vi "Cycle RGB Colors.vi"(3 "Magnitude":dbl, 4 "Cycle Speed":i32=5, 5 "Iteration":i32, 6 "Cycle Colors?":bool) -> (0 "Blue Value":u8, 1 "Green Value":u8, 2 "Red Value":u8)   [LabVIEW 2011, in "LabVIEW Interface for Arduino.lvlib"]
doc: "Cycles through RGB colors and outputs the appropriate Red Green and Blue values scaled by the specified Magnitude."
uses:
  LabVIEW Interface for Arduino.lvlib
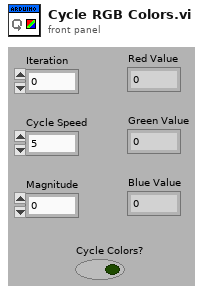
[diagram p1: front panel]
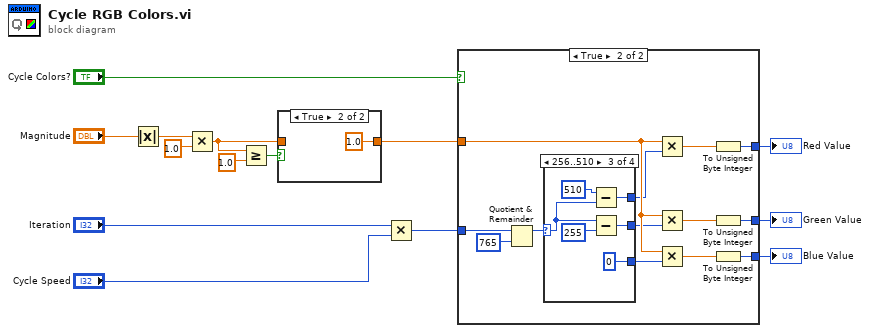
[diagram p0: block diagram]
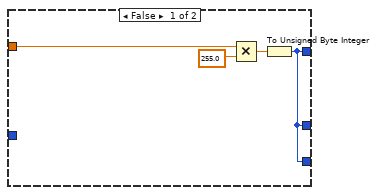
[diagram p2: hidden frame]
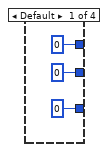
[diagram p3: hidden frame]
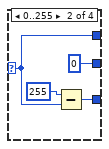
[diagram p4: hidden frame]
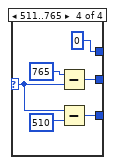
[diagram p5: hidden frame]
diagram:
  n1 = Absolute Value(x="Magnitude") -> (abs(x)=w1:dbl)
  n2 = Multiply(x=w1, y=1.0) -> (x*y=w5:dbl)
  n3 = Greater Or Equal?(x=w5, y=1.0) -> (x >= y?=w4:bool)
  n4 = case shown="True" w4 {
    tunnel: w5 -> [w15 _]
    tunnel: [w15 1.0 ("y")] -> w7
    frame False {
    }
    frame True {
    }
  }
  n5 = Multiply(x="Iteration", y="Cycle Speed") -> (x*y=w13:i32)
  n6 = case shown="True" "Cycle Colors?" {
    tunnel: w13 -> [_ w31]
    tunnel: w7 -> [w18 w30]
    tunnel: [w20 w23] -> w10
    tunnel: [w20 w22] -> w8
    tunnel: [w20 w21] -> w9
    frame False {
      n7 = Multiply(x=w18, y=255.0) -> (x*y=w17:dbl)
      n8 = To Unsigned Byte Integer(number=w17) -> (unsigned 8bit integer=w20:u8)
    }
    frame True {
      n9 = Quotient & Remainder(x=w31, y=765) -> (x-y*floor(x/y)=w33:i32)  [unwired: 1 out]
      n10 = case shown="256..510" w33 {
        selector: w33 -> [_ w40 w41 w48]
        tunnel: [0 ("y") w40 w44 0 ("y")] -> w29
        tunnel: [0 0 w45 w49] -> w28
        tunnel: [0 ("y") w38 u8 0 ("y") w50] -> w27
        frame Default {
        }
        frame 0..255 {
          n11 = Subtract(x=255, y=w40) -> (x-y=w38:i32)
        }
        frame 256..510 {
          n12 = Subtract(x=510 ("y"), y=w41) -> (x-y=w44:i32)
          n13 = Subtract(x=w41, y=255) -> (x-y=w45:i32)
        }
        frame 511..765 {
          n14 = Subtract(x=765, y=w48) -> (x-y=w49:i32)
          n15 = Subtract(x=w48, y=510) -> (x-y=w50:i32)
        }
      }
      n16 = Multiply(x=w30, y=w29) -> (x*y=w26:dbl)
      n17 = Multiply(x=w30, y=w28) -> (x*y=w25:dbl)
      n18 = Multiply(x=w30, y=w27) -> (x*y=w24:dbl)
      n19 = To Unsigned Byte Integer(number=w26) -> (unsigned 8bit integer=w21:u8)
      n20 = To Unsigned Byte Integer(number=w25) -> (unsigned 8bit integer=w22:u8)
      n21 = To Unsigned Byte Integer(number=w24) -> (unsigned 8bit integer=w23:u8)
    }
  }
  "Blue Value" <- w10
  "Red Value" <- w9
  "Green Value" <- w8
